vi "pythonDisplayImageTest.vi"() -> ()   [LabVIEW 2017]
uses:
  globalUtilities.vi
  dll/wormUtilities/x64/Release/wormUtilities.dll
panel:
  out "return type":dbl
  out "x-y":dbl format="%.9f"
  in  "stop 4":bool
  out "Intensity Graph":u16[][](graph)
  in  "stop 3":bool
  # "Arrays work only if they have size >1 (2 is fine). Dunno why."
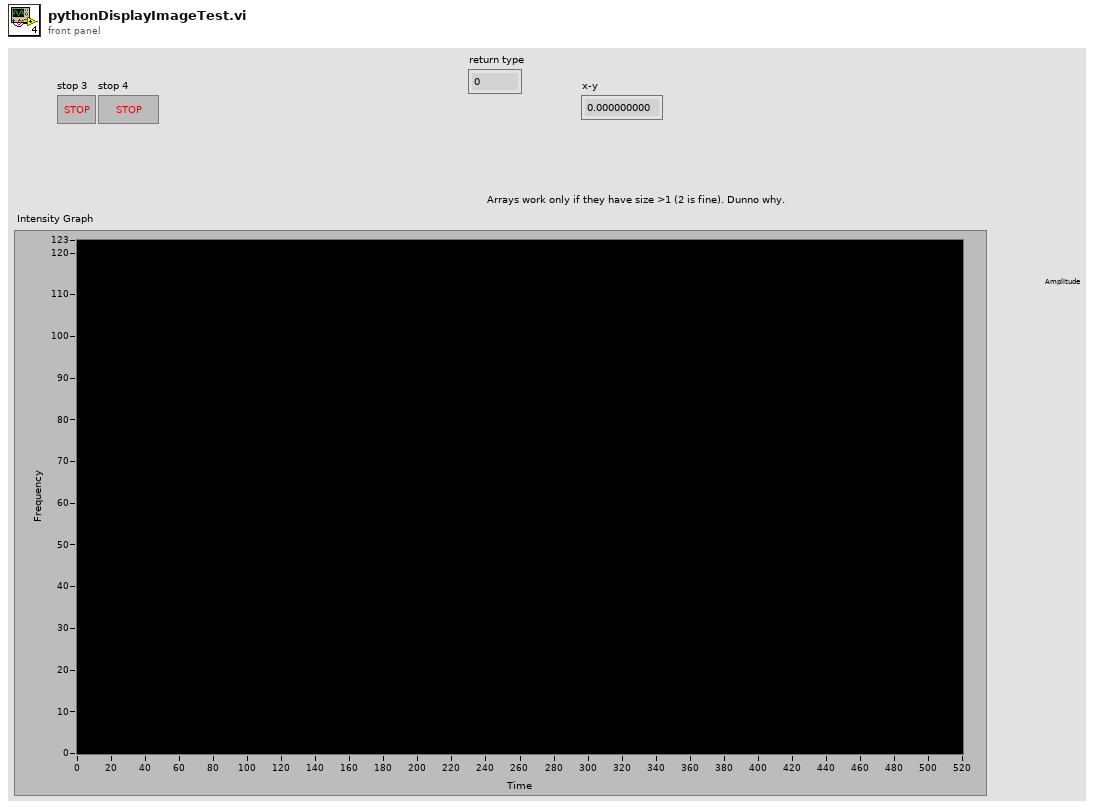
[diagram p1: front panel]
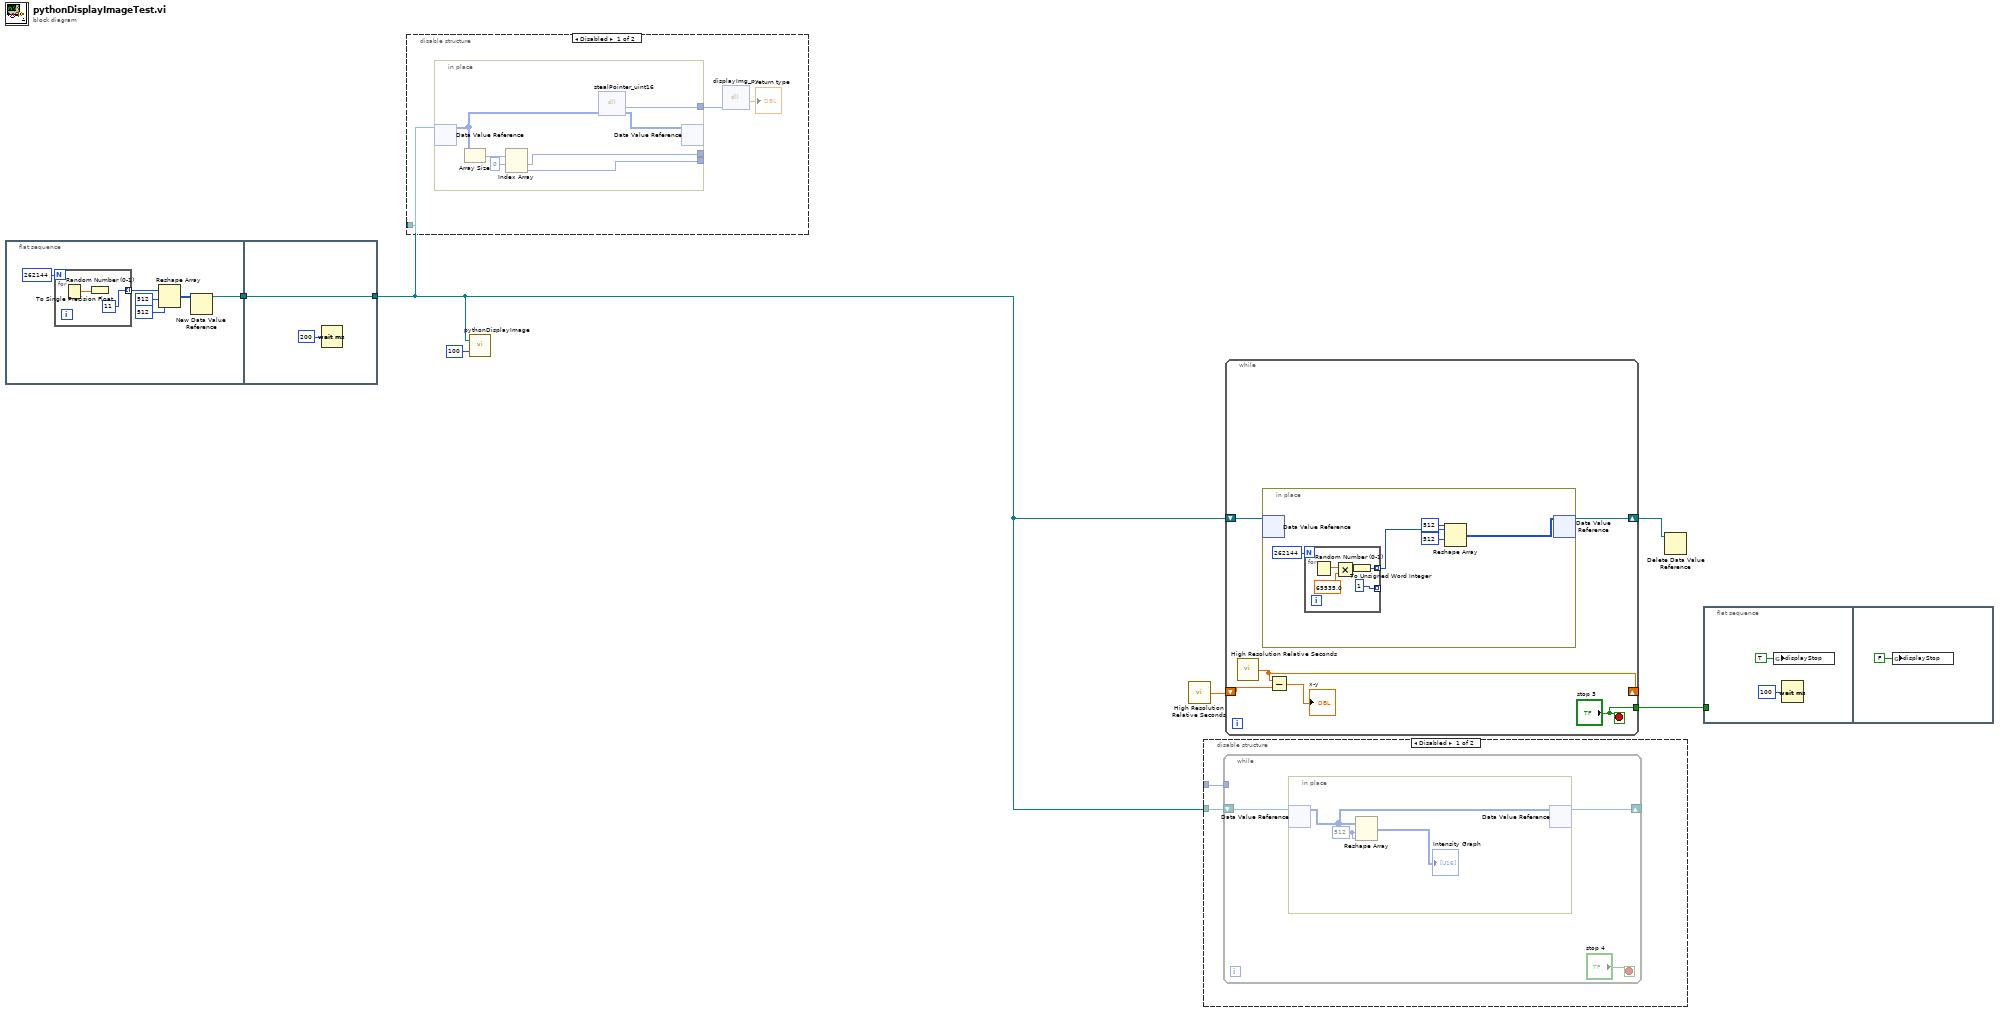
[diagram p0: block diagram]
diagram:
  n1 = flat-sequence {
    tunnel: [w7] -> w3
    tunnel: [w16] -> w2
    tunnel: w3 -> [w16]
    frame #0 {
      n2 = for {
        N: 262144 ("dimension size") -> [_]
        tunnel: [u16 11] -> w11 mode=indexing
        n3 = Random Number (0-1)() -> (number: 0 to 1=w14:dbl)
        n4 = To Single Precision Float(number=w14) -> ()  [unwired: 1 out]
      }
      n5 = Reshape Array(w11, 512 ("dimension size"), 512 ("dimension size")) -> (w8:u16[][])
      n6 = New Data Value Reference(data value=w8) -> (data value reference=w7:refnum<data-value>)  [unwired: 1 in, 1 out]
    }
    frame #1 {
      n7 = Wait (ms)(milliseconds to wait=u32 200) -> ()  [unwired: 1 out]
    }
  }
  n8 = disable-structure shown="Disabled" {
    disable-tunnel: w2 -> [w17 _]
    frame Disabled {
      n9 = in-place {
        in-place-border: [w26] -> w19
        in-place-border: [w23] -> _
        in-place-border: [w22] -> _
        n10 = in-place-dvr #1(w17) -> (w21:u16[][])  [unwired: 1 out]
        n11 = Array Size(array=w21) -> (size(s)=w25:i32[])
        n12 = Index Array(array=w25, index #1=0 ("index")) -> (element #1=w23:i32, element #2=w22:i32)  [unwired: 1 in]
        n13 = dll-call lib="C:/Users/francesco/dev/pump-probe/dll/wormUtilities/x64/Release/wormUtilities.dll" fn="stealPointer_uint16"("A"=w21) -> ("return type"=w26:i64, "A"=w20:u16[][])  [unwired: 3 in, 2 out]
        n14 = in-place-dvr #1(w20) -> ()  [unwired: 2 out]
      }
      n15 = dll-call lib="C:/Users/francesco/dev/pump-probe/dll/wormUtilities/x64/Release/wormUtilities.dll" fn="displayImg_py"("A"=w19) -> ("return type"=→"return type":dbl)  [unwired: 4 in, 2 out]
    }
    frame Enabled {
    }
  }
  n16 = call "pythonDisplayImage.vi"("refresh_time"=100, "image reference"=w2) -> ()  [unwired: 1 in]
  n17 = call <vilib>:"High Resolution Relative Seconds.vi"() -> ("relative seconds"=w5:dbl)
  n18 = disable-structure shown="Disabled" {
    disable-tunnel: _ -> [w28 _]
    disable-tunnel: w2 -> [w27 _]
    frame Disabled {
      n19 = while {
        shift-right: [w30] -> _
        shift-left: w27 -> [w31]
        tunnel: w28 -> [_]
        stop <- "stop 4" stop-if-true
        n20 = in-place {
          w34 = 512 ("dimension size")
          n21 = in-place-dvr #2(w31) -> (w32:u16[][])  [unwired: 1 out]
          n22 = Reshape Array(w32, w34, w34) -> (→"Intensity Graph":u16[][])
          n23 = in-place-dvr #2(w32) -> (w30:refnum<data-value>)  [unwired: 1 out]
        }
      }
    }
    frame Enabled {
    }
  }
  n24 = while {
    shift-right: [w36] -> _
    shift-left: w5 -> [w38]
    tunnel: ["stop 3"] -> w4
    shift-right: [w39] -> w6
    shift-left: w2 -> [w40]
    stop <- "stop 3" stop-if-true
    n25 = call <vilib>:"High Resolution Relative Seconds.vi"() -> ("relative seconds"=w36:dbl)
    n26 = in-place {
      n27 = in-place-dvr #3(w40) -> ()  [unwired: 2 out]
      n28 = for {
        N: 262144 ("dimension size") -> [_]
        tunnel: [w50] -> w44 mode=indexing
        tunnel: [u16 1] -> _ mode=indexing
        n29 = Random Number (0-1)() -> (number: 0 to 1=w48:dbl)
        n30 = Multiply(x=w48, y=65535.0) -> (x*y=w46:dbl)
        n31 = To Unsigned Word Integer(number=w46) -> (unsigned 16bit integer=w50:u16)
      }
      n32 = Reshape Array(w44, 512 ("dimension size"), 512 ("dimension size")) -> (w41:u16[][])
      n33 = in-place-dvr #3(w41) -> (w39:refnum<data-value>)  [unwired: 1 out]
    }
    n34 = Subtract(x=w36, y=w38) -> (x-y=→"x-y":dbl)
  }
  n35 = Delete Data Value Reference(data value reference=w6) -> ()  [unwired: 1 in, 2 out]
  n36 = flat-sequence {
    tunnel: w4 -> [_]
    frame #0 {
      n37 = global write "globalUtilities.vi" "displayStop"(TRUE ("generalStop")) -> ()
      n38 = Wait (ms)(milliseconds to wait=u32 100) -> ()  [unwired: 1 out]
    }
    frame #1 {
      n39 = global write "globalUtilities.vi" "displayStop"(FALSE ("generalStop")) -> ()
    }
  }
